vi "Sensor Init.vi"(1 "error in":errorcluster) -> (0 "error out":errorcluster)   [LabVIEW 2014]
panel:
  out "Calibrated Center Voltage Out":dbl
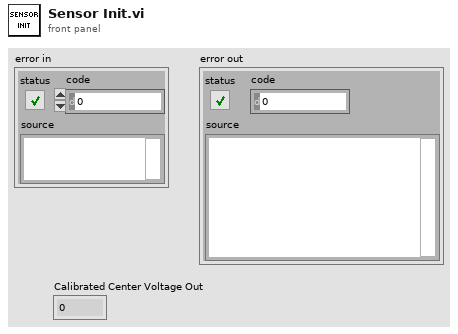
[diagram p1: front panel]
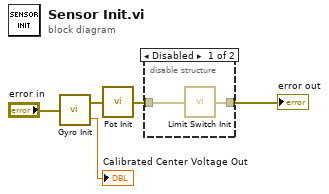
[diagram p0: block diagram]
diagram:
  n1 = call "Gyro Init.vi"("error in"="error in") -> ("error out"=w1:errorcluster, "Calibrated Center Voltage Out"=→"Calibrated Center Voltage Out":dbl)
  n2 = call "Pot Init.vi"("error in"=w1) -> ("error out"=w4:errorcluster)
  n3 = disable-structure shown="Disabled" {
    disable-tunnel: [w7 _] -> w5
    disable-tunnel: w4 -> [w6 _]
    frame Disabled {
      n4 = call "Limit Switch Init.vi"("error in"=w6) -> ("error out"=w7:errorcluster)
    }
    frame Enabled {
    }
  }
  "error out" <- w5
